vi "Lakeshore_monitor_2014 07 02.vi"(7 "Error In":errorcluster, 10 "VISA Resource (TPX)":refnum<visa-resource-name>="LakeShore336") -> (0 "Error Out":errorcluster, 1 "Outputs":T1 {"Heater 1 Output 2" format="%_3g"; "Heater 2 Output 1" format="%_3g"}, 2 "Inputs":T2 {"A:  Sample Stage" format="%_6g"; "B:  Rad Shield" format="%_6g"}, 3 "VISA Resource (TPX) Out":refnum<visa-resource-name>)   [LabVIEW 2012]
doc: "This .vi reads the current state of the front panel of the LakeShore temperature controller."
uses:
  Instrument Libraries/Lake Shore 336/Public/Data/Sensor Data (Single Reading).vi
  Instrument Libraries/Lake Shore 336/Lake Shore 336.lvlib
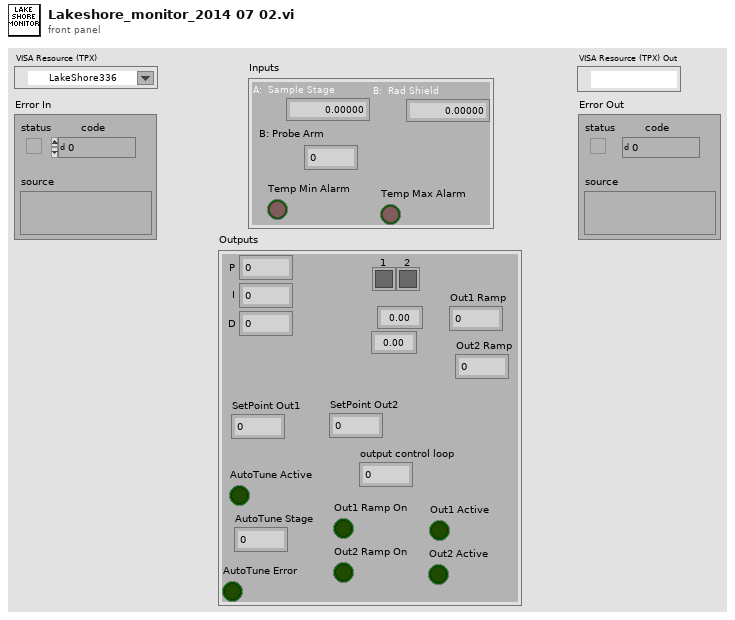
[diagram p1: front panel]
types:
  T1 = cluster{"P":dbl, "I":dbl, "D":dbl, "SetPoint Out1":dbl, "SetPoint Out2":dbl, "1":bool, "2":bool, "output control loop":dbl, "AutoTune Error":bool, "AutoTune Active":bool, "AutoTune Stage":dbl, "Out1 Active":bool, "Out1 Ramp On":bool, "Out2 Active":bool, "Out2 Ramp On":bool, "Heater 2 Output 1":dbl, "Heater 1 Output 2":dbl, "Out1 Ramp":dbl, "Out2 Ramp":dbl}
  T2 = cluster{"A:  Sample Stage":dbl, "B:  Rad Shield":dbl, "B: Probe Arm":dbl, "Temp Max Alarm":bool, "Temp Min Alarm":bool}
  T3 = cluster{"Sensor Data":dbl, "Sensor Data":dbl, "Sensor Data":dbl, "High Alarm Active?":bool, "Low Alarm Active?":bool}
  T4 = cluster{"Gain (P)":dbl, "Reset (I)":dbl, "Rate (D)":dbl, "Setpoint":dbl, "Setpoint":dbl, bool, bool, "Output's Control Loop":u16, "Tuning Error?":bool, "Tuning Active?":bool, "Stage Status":u16, "Ramping Active?":bool, "Ramping On?":bool, "Ramping Active?":bool, "Ramping On?":bool, "Output Value":dbl, "Output Value":dbl, "Ramp Rate":dbl, "Ramp Rate":dbl}
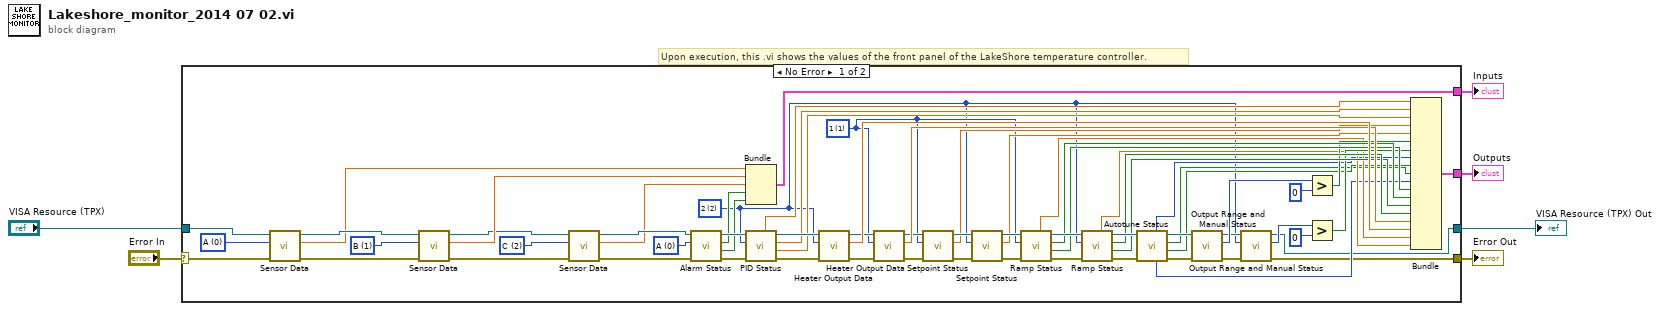
[diagram p0: block diagram]
diagram:
  # "Upon execution, this .vi shows the values of the front panel of the LakeShore temperature controller."
  n1 = case shown="No Error" "Error In" {
    selector: "Error In" -> [w19 w74]
    tunnel: [w25 w74] -> w6
    tunnel: "VISA Resource (TPX)" -> [w10 w73]
    tunnel: [w9 _] -> w3
    tunnel: [w8 _] -> w2
    tunnel: [w7 w73] -> w1
    frame No Error {
      w11 = u16 0 items=["A", "B", "C", "D"] ("Input (0:A)")
      w12 = u16 0 items=["A", "B", "C", "D"] ("Input (0:A)")
      w15 = u16 1 items=["A", "B", "C", "D"] ("Input (0:A)")
      w16 = u16 2 items=["A", "B", "C", "D"] ("Input (0:A)")
      w17 = u16 2 items=["1"=1, "2"=2] ("Output's Control Loop (1:1)")
      w18 = u16 1 items=["1"=1, "2"=2] ("Heater Output (1:1)")
      n2 = call-poly "Sensor Data.vi"("error in (no error)"=w19, "Input (0:A)"=w11, "VISA resource name"=w10) -> ("error out"=w69:errorcluster, "Sensor Data"=w64:dbl, "VISA resource name out"=w70:refnum<visa-resource-name>)  [unwired: 6 in]
      n3 = call-poly "Sensor Data.vi"("error in (no error)"=w69, "Input (0:A)"=w15, "VISA resource name"=w70) -> ("error out"=w20:errorcluster, "Sensor Data"=w63:dbl, "VISA resource name out"=w24:refnum<visa-resource-name>)  [unwired: 6 in]
      n4 = call-poly "Sensor Data.vi"("error in (no error)"=w20, "Input (0:A)"=w16, "VISA resource name"=w24) -> ("error out"=w21:errorcluster, "Sensor Data"=w22:dbl, "VISA resource name out"=w23:refnum<visa-resource-name>)  [unwired: 6 in]
      n5 = call "Alarm Status.vi"("error in (no error)"=w21, "Input (0:A)"=w12, "VISA resource name"=w23) -> ("error out"=w67:errorcluster, "Low Alarm Active?"=w61:bool, "High Alarm Active?"=w62:bool, "VISA resource name out"=w68:refnum<visa-resource-name>)  [unwired: 5 in]
      n6 = Bundle("Sensor Data"=w64, "Sensor Data"=w63, "Sensor Data"=w22, "High Alarm Active?"=w62, "Low Alarm Active?"=w61) -> (w9:T3)  [unwired: 1 in]
      n7 = call "PID Status.vi"("error in (no error)"=w67, "Output's Control Loop (1:1)"=w17, "VISA resource name"=w68) -> ("error out"=w65:errorcluster, "Rate (D)"=w58:dbl, "Reset (I)"=w59:dbl, "VISA resource name out"=w66:refnum<visa-resource-name>, "Gain (P)"=w60:dbl)  [unwired: 4 in]
      n8 = call "Heater Output Data.vi"("error in (no error)"=w65, "Heater Output (1:1)"=w17, "VISA resource name"=w66) -> ("error out"=w55:errorcluster, "Output Value"=w57:dbl, "VISA resource name out"=w56:refnum<visa-resource-name>)  [unwired: 6 in]
      n9 = call "Heater Output Data.vi"("error in (no error)"=w55, "Heater Output (1:1)"=w18, "VISA resource name"=w56) -> ("error out"=w50:errorcluster, "Output Value"=w54:dbl, "VISA resource name out"=w51:refnum<visa-resource-name>)  [unwired: 6 in]
      n10 = call "Setpoint Status.vi"("error in (no error)"=w50, "Output (1:1)"=w18, "VISA resource name"=w51) -> ("error out"=w53:errorcluster, "Setpoint"=w48:dbl, "VISA resource name out"=w52:refnum<visa-resource-name>)  [unwired: 6 in]
      n11 = call "Setpoint Status.vi"("error in (no error)"=w53, "Output (1:1)"=w17, "VISA resource name"=w52) -> ("error out"=w72:errorcluster, "Setpoint"=w49:dbl, "VISA resource name out"=w71:refnum<visa-resource-name>)  [unwired: 6 in]
      n12 = call "Ramp Status.vi"("error in (no error)"=w72, "Output's Control Loop (1:1)"=w18, "VISA resource name"=w71) -> ("error out"=w46:errorcluster, "Ramping Active?"=w40:bool, "Ramping On?"=w41:bool, "VISA resource name out"=w47:refnum<visa-resource-name>, "Ramp Rate"=w33:dbl)  [unwired: 4 in]
      n13 = call "Ramp Status.vi"("error in (no error)"=w46, "Output's Control Loop (1:1)"=w17, "VISA resource name"=w47) -> ("error out"=w44:errorcluster, "Ramping Active?"=w42:bool, "Ramping On?"=w43:bool, "VISA resource name out"=w45:refnum<visa-resource-name>, "Ramp Rate"=w32:dbl)  [unwired: 4 in]
      n14 = call "Autotune Status.vi"("error in (no error)"=w44, "VISA resource name"=w45) -> ("error out"=w30:errorcluster, "Tuning Error?"=w28:bool, "Tuning Active?"=w27:bool, "VISA resource name out"=w31:refnum<visa-resource-name>, "Stage Status"=w26:u16, "Output's Control Loop"=w29:u16)  [unwired: 4 in]
      n15 = call "Output Range and Manual Status.vi"("error in (no error)"=w30, "VISA resource name"=w31) -> ("error out"=w37:errorcluster, "Range (0:Off)"=w39:u16, "VISA resource name out"=w38:refnum<visa-resource-name>)  [unwired: 6 in, 1 out]
      n16 = call "Output Range and Manual Status.vi"("error in (no error)"=w37, "Output (1:1)"=w17, "VISA resource name"=w38) -> ("error out"=w25:errorcluster, "Range (0:Off)"=w36:u16, "VISA resource name out"=w7:refnum<visa-resource-name>)  [unwired: 5 in, 1 out]
      n17 = Greater?(x=w39, y=u16 0) -> (0:w35:bool)
      n18 = Greater?(x=w36, y=u16 0) -> (0:w34:bool)
      n19 = Bundle("Gain (P)"=w60, "Reset (I)"=w59, "Rate (D)"=w58, "Setpoint"=w48, "Setpoint"=w49, w35, w34, "Output's Control Loop"=w29, "Tuning Error?"=w28, "Tuning Active?"=w27, "Stage Status"=w26, "Ramping Active?"=w40, "Ramping On?"=w41, "Ramping Active?"=w42, "Ramping On?"=w43, "Output Value"=w54, "Output Value"=w57, "Ramp Rate"=w33, "Ramp Rate"=w32) -> (w8:T4)  [unwired: 1 in]
    }
    frame Error {
    }
  }
  "Error Out" <- w6
  "Inputs" <- w3
  "Outputs" <- w2
  "VISA Resource (TPX) Out" <- w1
